vi "OpenConnection.vi"(8 "error in (no error)":errorcluster, 11 "object in":refnum<class "RS232.lvclass">) -> (0 "error out":errorcluster, 3 "object out":refnum<class "RS232.lvclass">)   [LabVIEW 2019, in "RS232.lvclass"]
uses:
  RS232.lvclass
  <vilib>/Instr/_visa.llb/VISA Flush IO Buffer Mask.ctl
  RS232.lvclass/RS232.ctl
  <vilib>/Instr/_visa.llb/VISA Configure Serial Port (Instr).vi
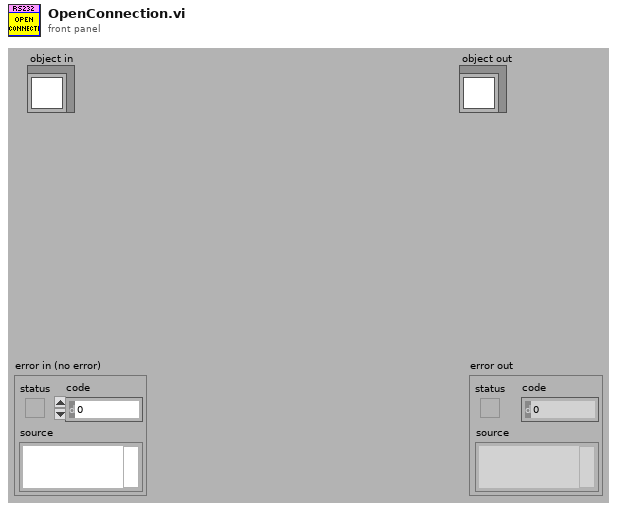
[diagram p1: front panel]
types:
  T1 = typedef "VISA Flush IO Buffer Mask.ctl" = u16
  T2 = typedef "RS232.lvclass/SettingCtrl.ctl" = cluster{"ComPort":string}
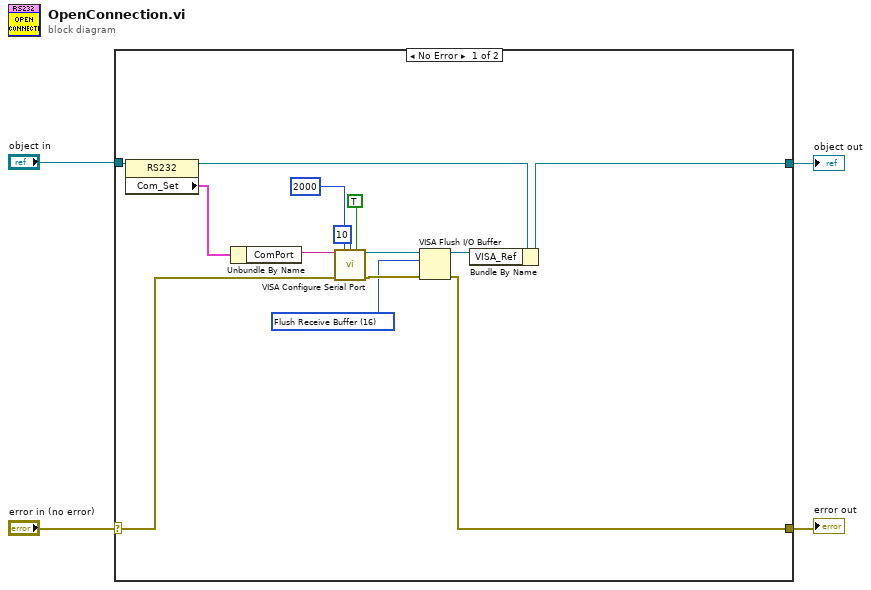
[diagram p0: block diagram]
diagram:
  n1 = case shown="No Error" "error in (no error)" {
    selector: "error in (no error)" -> [w11 w20]
    tunnel: [w6 w20] -> w3
    tunnel: [w17 w19] -> w1
    tunnel: "object in" -> [w18 w19]
    frame No Error {
      w5 = T1 16 items=["Flush Receive Buffer"=16, "Write Transmit Buffer to Device"=32, "Flush Receive Buffer (No I/O)"=64, "Flush Transmit Buffer"=128] ("Mask")
      n2 = property class="RS232"(reference=w18) -> (reference out=w16:refnum<class "RS232.lvclass">, "Com_Set"=w15:T2)  [unwired: 1 in, 1 out]
      n3 = Unbundle By Name(w15) -> ("ComPort"=w14:string)
      n4 = call-poly "VISA Configure Serial Port"("VISA resource name"=w14, "timeout (10sec)"=u32 2000, "termination char\n(0xA = '\\n' = LF)"=u8 10 ("termination char\n(0xA = '\\n' = LF)"), "Enable Termination\nChar (T)"=TRUE ("Enable Termination\nChar (T)"), "error in (no error)"=w11) -> ("VISA resource name out"=w10:refnum<visa-resource-name>, "error out"=w7:errorcluster)  [unwired: 9 in]
      n5 = VISA Flush I/O Buffer(VISA resource name=w10, mask (16)=w5, error in (no error)=w7) -> (VISA resource name out=w8:refnum<visa-resource-name>, error out=w6:errorcluster)
      n6 = Bundle By Name(cluster=w16, "VISA_Ref"=w8) -> (w17:refnum<class "RS232.lvclass">)
    }
    frame Error {
    }
  }
  "error out" <- w3
  "object out" <- w1
